vi "Get Msg Attributes.vi"(11 "Actor Last Ack Msg Strategy in":refnum<class "Actor Last Ack Msg Strategy.lvclass">) -> (1 "Nested Error":errorcluster, 2 "Nested Actor":refnum<class "Actor.lvclass">)   [LabVIEW 2021, in "Actor Last Ack.lvlib" / "Actor Last Ack Msg Strategy.lvclass"]
uses:
  Actor Last Ack Msg Strategy.lvclass
  LVCAM/Actor/Actor.lvclass
  Actor Last Ack Msg Strategy.lvclass/Actor Last Ack Msg Strategy.ctl
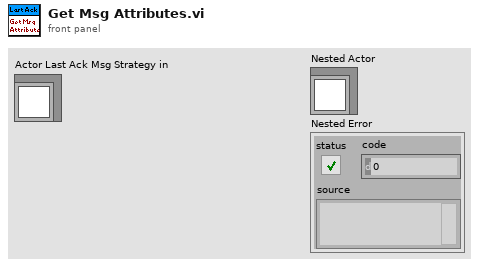
[diagram p1: front panel]
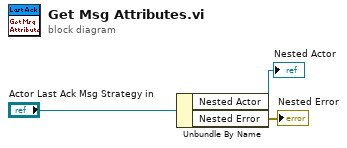
[diagram p0: block diagram]
diagram:
  n1 = Unbundle By Name("Actor Last Ack Msg Strategy in") -> ("Nested Actor"=→"Nested Actor":refnum<class "Actor.lvclass">, "Nested Error"=→"Nested Error":errorcluster)
